vi "Name.vi"(7 "Address":string, 8 "Error In":errorcluster) -> (0 "Error Out":errorcluster)   [LabVIEW 2018, in "Tests.lvlib" / "Known Host.lvlib"]
uses:
  Known Host.lvlib
  src/Toolkit/Known Host/Known Host.lvclass/Known Host.ctl
  src/Toolkit/SSH/SSH.lvclass/SSH.ctl
  src/Toolkit/SSH/Utility/Read Shared Library.vi
  src/Toolkit/Known Host/Support/Name Length.vi
  src/Toolkit/Support/Check Status.vi
  <vilib>/addons/_JKI Toolkits/Caraya/classes/Test/Test.lvclass
  <vilib>/addons/_JKI Toolkits/Caraya/classes/Assert/Assert.lvclass
  src/Toolkit/Known Host/Known Host.lvclass
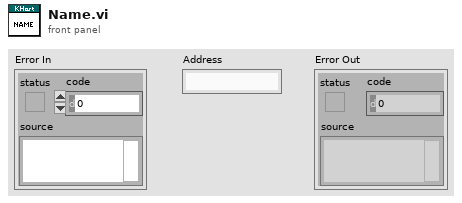
[diagram p1: front panel]
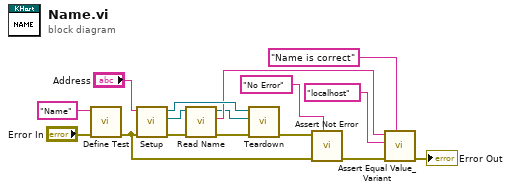
[diagram p0: block diagram]
diagram:
  n1 = call <vilib>:"Define Test.vi"("error in (no error)"="Error In", "Label (VI Title)"="Name") -> ("error out"=w12:errorcluster)  [unwired: 9 in]
  n2 = call "Setup.vi"("Error In"=w12, "Address"="Address") -> ("Error Out"=w10:errorcluster, "Known Host"=w2:refnum<class "Known Host.lvclass">, "Known Hosts"=w8:refnum<class "Known Hosts.lvclass">)  [unwired: 7 in]
  n3 = call "Read Name.vi"("Error In"=w10, "Known Host In"=w2) -> ("Error Out"=w9:errorcluster, "Name"=w4:string, "Known Host Out"=w1:refnum<class "Known Host.lvclass">)  [unwired: 7 in]
  n4 = call "Teardown.vi"("Error In"=w9, "Known Host"=w1, "Known Hosts"=w8) -> ("Error Out"=w7:errorcluster)  [unwired: 8 in]
  n5 = call <vilib>:"Assert Not Error.vi"("Label"="No Error", "error in (no error)"=w12, "Not Error?"=w7) -> ("error out"=w13:errorcluster)  [unwired: 8 in]
  n6 = call <vilib>:"Assert Equal Value_Variant.vi"("Label"="Name is correct", "error in (no error)"=w13, "Y"="localhost" ("Name"), "X"=w4) -> ("error out"=→"Error Out":errorcluster)  [unwired: 7 in]
